vi "FPGA_AnalogTriggerReadConfiguration.vi"(8 "error in (no error)":errorcluster, 11 "AnalogTriggerDevRef":T3) -> (0 "error out":errorcluster, 2 "AnalogTriggerSource":T1={"Channel"=enum."AI 1", "Averaged"=FALSE, "Filter"=FALSE}, 3 "AnalogTriggerDevRef":T3)   [LabVIEW 2017]
uses:
  <vilib>/Rock Robotics/SystemInterfaces/AnalogTrigger/FPGA_AnalogTriggerDevRef.ctl
  <vilib>/Rock Robotics/SystemInterfaces/AnalogTrigger/FPGA_AnalogTriggerIndex.ctl
  <vilib>/Rock Robotics/SystemInterfaces/AnalogTrigger/FPGA_AnalogTriggerSource.ctl
  <vilib>/Rock Robotics/SystemInterfaces/AI/FPGA_AIChannel.ctl
  <vilib>/Rock Robotics/SystemInterfaces/System/FPGA_SystemFPGA Ref Global.vi
  <vilib>/Utility/error.llb/Error Cluster From Error Code.vi
  <vilib>/rvi/errors/niLvFpgaAdjustHostInterfaceError.vi
  <vilib>/rvi/interface/nirviReadWriteControl/nirviReadWriteControl.xnode
  <vilib>/Rock Robotics/SystemInterfaces/System/FPGA_SystemFRC FPGA Ref.ctl
  NiFpgaLv.dll
  <vilib>/rvi/interface/Simulation/niFpgaSimulationCallBeginRW.vi
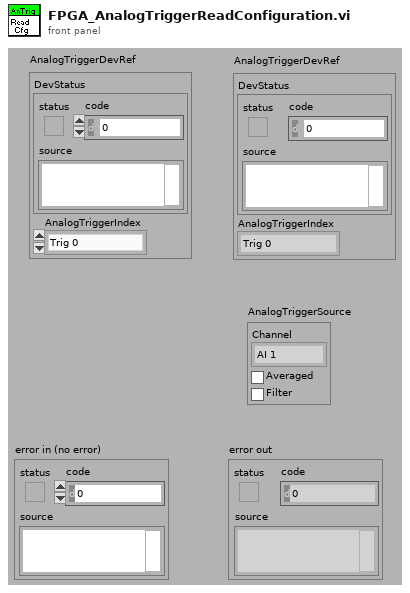
[diagram p1: front panel]
types:
  T1 = typedef "FPGA_AnalogTriggerSource.ctl" = cluster{"Channel":T2, "Averaged":bool, "Filter":bool}
  T2 = typedef "FPGA_AIChannel.ctl" = enum8{"AI 0", "AI 1", "AI 2", "AI 3", "AI MXP 0", "AI MXP 1", "AI MXP 2", "AI MXP 3", "Invalid"}
  T3 = typedef "FPGA_AnalogTriggerDevRef.ctl" = cluster{"DevStatus":errorcluster, "AnalogTriggerIndex":T4}
  T4 = typedef "FPGA_AnalogTriggerIndex.ctl" = enum8{"Trig 0", "Trig 1", "Trig 2", "Trig 3", "Trig 4", "Trig 5", "Trig 6", "Trig 7", "Invalid"}
  T5 = typedef "FPGA_SystemFRC FPGA Ref.ctl" = refnum<k20>
  T6 = cluster{"Channel":fxp<+,3,3>, "Averaged":bool, "Filter":bool, "FloatingRollover":bool, "RolloverLimit":fxp<+/-,8,12>}
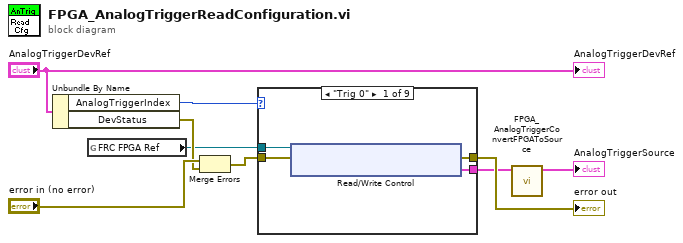
[diagram p0: block diagram]
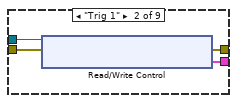
[diagram p2: hidden frame]
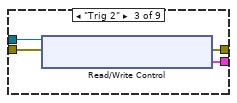
[diagram p3: hidden frame]
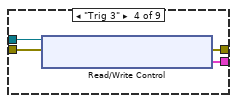
[diagram p4: hidden frame]
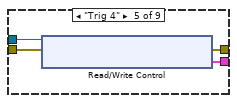
[diagram p5: hidden frame]
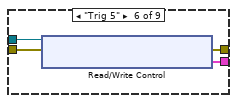
[diagram p6: hidden frame]
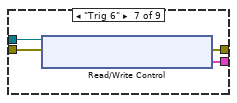
[diagram p7: hidden frame]
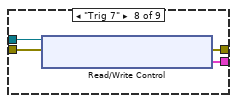
[diagram p8: hidden frame]
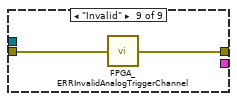
[diagram p9: hidden frame]
diagram:
  n1 = Unbundle By Name("AnalogTriggerDevRef") -> ("AnalogTriggerIndex"=w5:T4, "DevStatus"=w3:errorcluster)
  n2 = global read "FPGA_SystemFPGA Ref Global.vi" "FRC FPGA Ref"() -> (w1:T5)
  n3 = Merge Errors("error in (no error)", w3) -> (w2:errorcluster)
  n4 = case shown="\"Trig 0\"" w5 {
    tunnel: w1 -> [w12 w17 w21 w25 w29 w33 w37 w41 _]
    tunnel: w2 -> [w13 w16 w20 w24 w28 w32 w36 w40 w43]
    tunnel: [w11 w15 w19 w23 w27 w31 w35 w39 w42] -> w8
    tunnel: [w10 w14 w18 w22 w26 w30 w34 w38 _] -> w4
    frame "Trig 0" {
      n5 = xnode "Read/Write Control"("FPGA VI Reference In"=w12, "error in"=w13) -> ("error out"=w11:errorcluster, "AnalogTrigger0.SourceSelect"=w10:T6)  [unwired: 1 out]
    }
    frame "Trig 1" {
      n6 = xnode "Read/Write Control"("FPGA VI Reference In"=w17, "error in"=w16) -> ("error out"=w15:errorcluster, "AnalogTrigger1.SourceSelect"=w14:T6)  [unwired: 1 out]
    }
    frame "Trig 2" {
      n7 = xnode "Read/Write Control"("FPGA VI Reference In"=w21, "error in"=w20) -> ("error out"=w19:errorcluster, "AnalogTrigger2.SourceSelect"=w18:T6)  [unwired: 1 out]
    }
    frame "Trig 3" {
      n8 = xnode "Read/Write Control"("FPGA VI Reference In"=w25, "error in"=w24) -> ("error out"=w23:errorcluster, "AnalogTrigger3.SourceSelect"=w22:T6)  [unwired: 1 out]
    }
    frame "Trig 4" {
      n9 = xnode "Read/Write Control"("FPGA VI Reference In"=w29, "error in"=w28) -> ("error out"=w27:errorcluster, "AnalogTrigger4.SourceSelect"=w26:T6)  [unwired: 1 out]
    }
    frame "Trig 5" {
      n10 = xnode "Read/Write Control"("FPGA VI Reference In"=w33, "error in"=w32) -> ("error out"=w31:errorcluster, "AnalogTrigger5.SourceSelect"=w30:T6)  [unwired: 1 out]
    }
    frame "Trig 6" {
      n11 = xnode "Read/Write Control"("FPGA VI Reference In"=w37, "error in"=w36) -> ("error out"=w35:errorcluster, "AnalogTrigger6.SourceSelect"=w34:T6)  [unwired: 1 out]
    }
    frame "Trig 7" {
      n12 = xnode "Read/Write Control"("FPGA VI Reference In"=w41, "error in"=w40) -> ("error out"=w39:errorcluster, "AnalogTrigger7.SourceSelect"=w38:T6)  [unwired: 1 out]
    }
    frame "Invalid" {
      n13 = call <vilib>:"FPGA_ERRInvalidAnalogTriggerChannel.vi"("error in (no error)"=w43) -> ("error out"=w42:errorcluster)
    }
  }
  "error out" <- w8
  n14 = call <vilib>:"FPGA_AnalogTriggerConvertFPGAToSource.vi"("FPGASourceType"=w4) -> ("AnalogTriggerSource"=→"AnalogTriggerSource":T1)  [unwired: 10 out]
  "AnalogTriggerDevRef" <- "AnalogTriggerDevRef"
